vi "Set_Trigger_PassThrough_Disable.vi"(8 "error in (no error)":errorcluster, 11 ".NET Reference in":refnum<k24>) -> (0 "error out":errorcluster, 3 "Reference  out":refnum<k24>)   [LabVIEW 2017]
uses:
  C:/Users/Ssantec_Test/Documents/Installment_DLL_Sample_Labview_20211104/DLL/x86/InstrumentDLL.dll
  DLL/x86/InstrumentDLL.dll
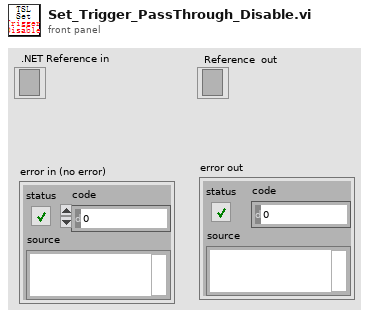
[diagram p1: front panel]
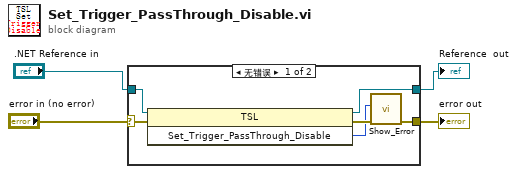
[diagram p0: block diagram]
diagram:
  n1 = case shown="无错误" "error in (no error)" {
    selector: "error in (no error)" -> [w5 w12]
    tunnel: ".NET Reference in" -> [w10 w11]
    tunnel: [w9 w11] -> w3
    tunnel: [w6 w12] -> w2
    frame No Error {
      n2 = invoke on="调用节点" class="TSL" method="Set_Trigger_PassThrough_Disable"(reference=w10, error in=w5) -> (reference out=w9:refnum<k24>, error out=w8:errorcluster, "Set_Trigger_PassThrough_Disable"=w7:i32)  [unwired: 1 in]
      n3 = call "Show_Error.vi"("error in (no error)"=w8, "Error"=w7) -> ("error out"=w6:errorcluster)  [unwired: 9 in]
    }
    frame Error {
    }
  }
  "Reference  out" <- w3
  "error out" <- w2
